vi "RT Loop - FPGA FIFO Read.vi"(8 "error in (no error)":errorcluster {"code" format="Error %.0f"}, 11 "FPGA VI Reference In":refnum<k20>) -> (0 "error out":errorcluster {"code" format="Error %.0f"}, 3 "Data Out":u16[][](array[numeric]))   [LabVIEW 2018]
uses:
  <vilib>/Utility/error.llb/Error Cluster From Error Code.vi
  <vilib>/rvi/errors/niLvFpgaAdjustHostInterfaceError.vi
  <vilib>/rvi/interface/nirviMethod/nirviMethod.xnode
  <vilib>/FPGAPlugInAG/Dynamic/niLvFpga_ReadFifo_Dynamic.vi
  <vilib>/rvi/errors/niLvFpgaMergeErrorWithErrorCode.vi
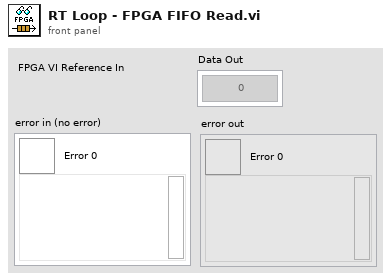
[diagram p1: front panel]
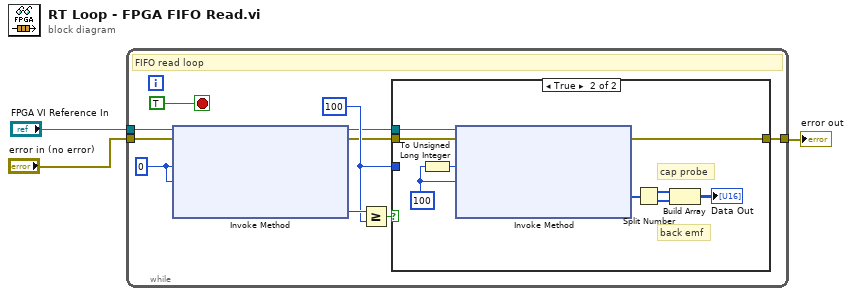
[diagram p0: block diagram]
diagram:
  n1 = while {
    tunnel: "FPGA VI Reference In" -> [w13]
    tunnel: "error in (no error)" -> [w7]
    tunnel: [w5] -> w3
    stop <- TRUE stop-if-true
    w10 = u32 100 ("Number of Elements 2")
    w6 = u32 0 ("Number of Elements")
    # "FIFO read loop"
    n2 = xnode "Invoke Method"("FPGA VI Reference In"=w13, "error in"=w7, "Number of Elements"=w6, "Timeout (ms)"=w6) -> ("FPGA VI Reference Out"=w9:refnum<k20>, "error out"=w8:errorcluster, "Elements Remaining"=w11:u32)  [unwired: 1 out]
    n3 = Greater Or Equal?(x=w11, y=w10) -> (x >= y?=w12:bool)
    n4 = case shown="True" w12 {
      tunnel: w10 -> [_ _]
      tunnel: w9 -> [_ w23]
      tunnel: w8 -> [w14 w22]
      tunnel: [w14 w21] -> w5
      frame False {
      }
      frame True {
        w20 = 100 ("Timeout (ms)")
        # "back emf"
        # "cap probe"
        n5 = To Unsigned Long Integer(number=w20) -> (unsigned 32bit integer=w19:u32)
        n6 = xnode "Invoke Method"("FPGA VI Reference In"=w23, "error in"=w22, "Number of Elements"=w19, "Timeout (ms)"=w20) -> ("error out"=w21:errorcluster, "Data"=w15:u32[])  [unwired: 2 out]
        n7 = Split Number(x=w15) -> (hi(x)=w18:u16[], lo(x)=w17:u16[])
        n8 = Build Array(w18, w17) -> (→"Data Out":u16[][])
      }
    }
  }
  "error out" <- w3
